vi "mapAngleToContrSubVi.vi"(0 "angleIn (rad)":dbl(knob) scale=-180.0..180.0) -> (3 "angleOut (rad)":dbl)   [LabVIEW 2011]
uses:
  <vilib>/imath/engines/lvmath2/RunTimeEngine/BuiltInFunctions/rem/NIMS_rem_no checks.vi
  <instcachedir>/0/NIMS_rem_no checks_8A14A2E4DF484AE391F841C42148F124.lvgen/NIMS_rem_no checks_8A14A2E4DF484AE391F841C42148F124_000.vi
  <vilib>/imath/engines/lvmath2/RunTimeEngine/BuiltInFunctions/abs/NIMS_abs(signed).vi
  <instcachedir>/0/NIMS_abs(signed)_C4FCB8E6058B49B797C7C8D53CA5F6EC.lvgen/NIMS_abs(signed)_C4FCB8E6058B49B797C7C8D53CA5F6EC_000.vi
  <vilib>/imath/engines/lvmath2/RunTimeEngine/NodeEndStatement/NIMS_NodeEndStatement_Output.vi
  <instcachedir>/0/NIMS_NodeEndStatement_Output_53EC0D466D134D7ABD903AC30B43404B.lvgen/NIMS_NodeEndStatement_Output_53EC0D466D134D7ABD903AC30B43404B_001.vi
  <vilib>/imath/engines/lvmath2/RunTimeEngine/ErrorHandling/NIMS_Finalize Error.vi
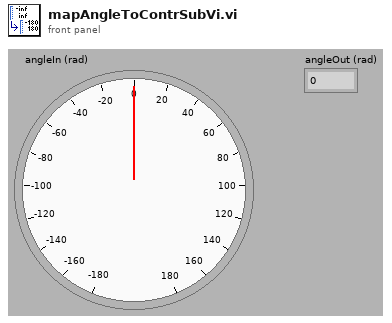
[diagram p1: front panel]
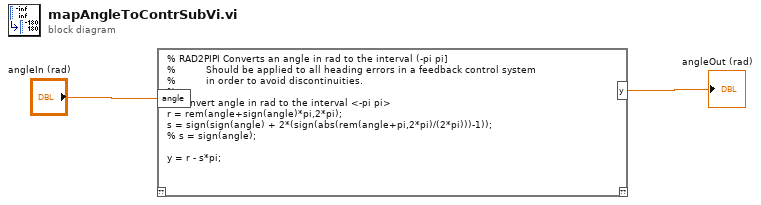
[diagram p0: block diagram]
diagram:
  n1 = mathscript code="% RAD2PIPI Converts an angle in rad to the interval (-pi pi]\n%          Should be applied to all heading errors in a feedback control system\n%          in order to avoid discontinuities.\n%\n% convert angle in rad to the interval <-pi pi> \nr = rem(angle+sign(angle)*pi,2*pi);\ns = sign(sign(angle) + 2*(sign(abs(rem(angle+pi,2*pi)/(2*pi)))-1));\n% s = sign(angle);\n\ny = r - s*pi;"("angle"="angleIn (rad)") -> ("y"=→"angleOut (rad)":dbl)  [unwired: 1 in, 1 out]
